vi "convert_ring_command.vi"(8 "error in (no error)":errorcluster, 10 "BD Ring Text":string="\n\nPOS\n\nNEG\nACT\n", 11 "Instrument Command":string=":CALC:CHP:MARK:MODE %s;") -> (0 "error out":errorcluster, 3 "Ring CMD":string=":CALC:CHP:MARK:MODE POS;\r:CALC:CHP:MARK:MODE DELT;\r:CALC:CHP:MARK:MODE OFF;\r")   [LabVIEW 2018]
uses:
  <vilib>/regexp/Match Regular Expression.xnode
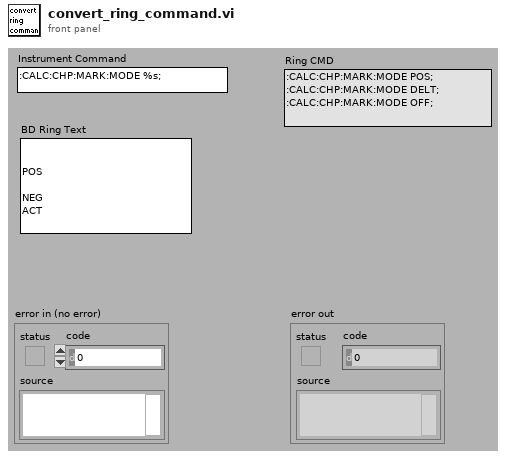
[diagram p1: front panel]
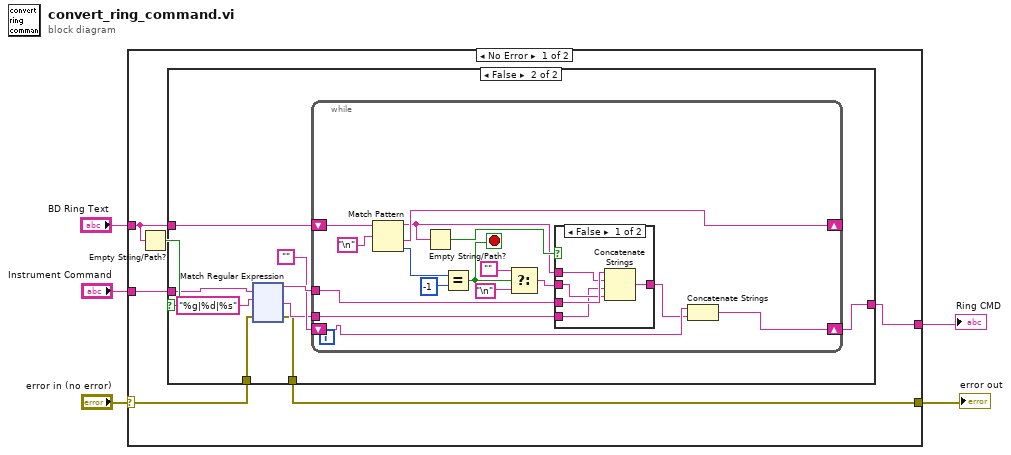
[diagram p0: block diagram]
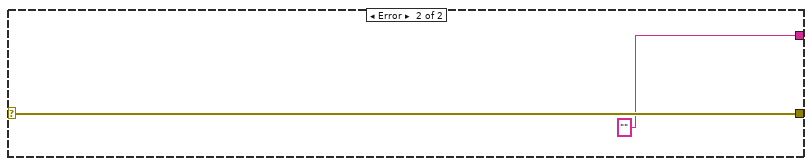
[diagram p4: hidden frame]
diagram:
  n1 = case shown="No Error" "error in (no error)" {
    selector: "error in (no error)" -> [w7 w157]
    tunnel: "Instrument Command" -> [w11 _]
    tunnel: [w10 "" ("Instrument Command")] -> w4
    tunnel: "BD Ring Text" -> [w9 _]
    tunnel: [w6 w157] -> w1
    frame No Error {
      n2 = Empty String/Path?(string/path=w9) -> (empty?=w8:bool)
      n3 = case shown="False" w8 {
        tunnel: w11 -> [w13 w16]
        tunnel: [w13 w19] -> w10
        tunnel: w9 -> [_ w18]
        tunnel: w7 -> [w12 w15]
        tunnel: [w12 w14] -> w6
        frame True {
        }
        frame False {
          n4 = xnode "Match Regular Expression"("input string"=w16, "regular expression"="%g|%d|%s", "error in"=w15) -> ("before match"=w21:string, "after match"=w17:string, "error out"=w14:errorcluster)  [unwired: 2 in, 3 out]
          n5 = while {
            shift-right: [w148] -> _
            shift-left: w18 -> [w149]
            tunnel: w21 -> [w144]
            shift-right: [w141] -> w19
            shift-left: "" -> [w142]
            tunnel: w17 -> [w134]
            stop <- w137 stop-if-true
            n6 = Match Pattern(string=w149, regular expression="\n") -> (before substring=w143:string, after substring=w148:string, offset past match=w147:i32)  [unwired: 1 in, 1 out]
            n7 = Empty String/Path?(string/path=w143) -> (empty?=w145:bool)
            n8 = Equal?(x=w147, y=-1) -> (x = y?=w137:bool)
            n9 = Select(t="", s=w137, f="\n") -> (s? t:f=w136:string)
            n10 = case shown="False" w145 {
              tunnel: w144 -> [w154 _]
              tunnel: w143 -> [w153 _]
              tunnel: [w152 w155] -> w140
              tunnel: w136 -> [w151 w155]
              tunnel: w134 -> [w150 _]
              frame False {
                n11 = Concatenate Strings(w154, w153, w150, w151) -> (w152:string)
              }
              frame True {
              }
            }
            n12 = Concatenate Strings(w142, w140) -> (w141:string)
          }
        }
      }
    }
    frame Error {
    }
  }
  "Ring CMD" <- w4
  "error out" <- w1
